vi "SpreadsheetRead.vi"() -> (0 "Output Cluster":cluster{"Y Array":dbl[], "X Array":dbl[]})   [LabVIEW 2014]
uses:
  <vilib>/Utility/file.llb/Read From Spreadsheet File (DBL).vi
panel:
  out "XY Graph":cluster{"all rows":dbl[], "all rows":dbl[]}(graph)
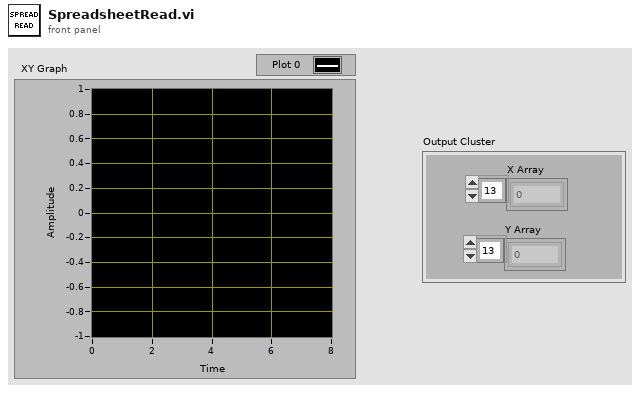
[diagram p1: front panel]
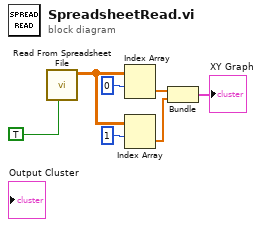
[diagram p0: block diagram]
diagram:
  n1 = call-poly <vilib>:"Read From Spreadsheet File.vi"("transpose (no:F)"=TRUE) -> ("all rows"=w5:dbl[][])  [unwired: 6 in, 4 out]
  n2 = Index Array(array=w5, index (row)=0) -> (element=w3:dbl[])  [unwired: 1 in]
  n3 = Index Array(array=w5, index (row)=1) -> (element=w2:dbl[])  [unwired: 1 in]
  n4 = Bundle("all rows"=w3, "all rows"=w2) -> (→"XY Graph":cluster{"all rows":dbl[], "all rows":dbl[]})  [unwired: 1 in]
